vi "Joystick Driver Controls.vi"(4 "Shift Value":T1, 7 "X":dbl, 11 "Y":dbl) -> (2 "Y":dbl, 3 "X":dbl)   [LabVIEW 2016]
uses:
  <vilib>/Rock Robotics/WPI/Solenoid/WPI_SolenoidValue.ctl
  <vilib>/Rock Robotics/Network Tables/NT Read Number.vi
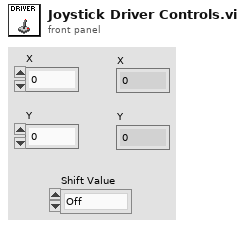
[diagram p1: front panel]
types:
  T1 = typedef "WPI_SolenoidValue.ctl" = enum16{"Off", "On", "Forward", "Reverse"}
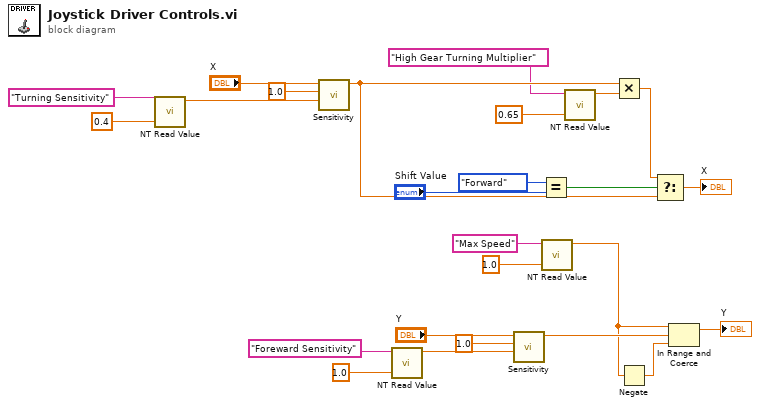
[diagram p0: block diagram]
diagram:
  n1 = call-poly <vilib>:"NT Read Value.vi"("Default Value"=0.4, "Name"="Turning Sensitivity") -> ("Numeric"=w7:dbl)  [unwired: 8 in, 1 out]
  n2 = call "Sensitivity.vi"("Power (z)"=w7, "Sensitivity (a)"=1.0, "Input"="X") -> ("Output"=w20:dbl)  [unwired: 8 in]
  n3 = call-poly <vilib>:"NT Read Value.vi"("Default Value"=1.0, "Name"="Foreward Sensitivity") -> ("Numeric"=w5:dbl)  [unwired: 8 in, 1 out]
  n4 = call "Sensitivity.vi"("Power (z)"=w5, "Sensitivity (a)"=1.0, "Input"="Y") -> ("Output"=w23:dbl)  [unwired: 8 in]
  n5 = Equal?(x=WPI_SolenoidValue."Forward", y="Shift Value") -> (x = y?=w15:bool)
  n6 = call-poly <vilib>:"NT Read Value.vi"("Default Value"=1.0, "Name"="Max Speed") -> ("Numeric"=w1:dbl)  [unwired: 8 in, 1 out]
  n7 = call-poly <vilib>:"NT Read Value.vi"("Default Value"=0.65, "Name"="High Gear Turning Multiplier") -> ("Numeric"=w10:dbl)  [unwired: 8 in, 1 out]
  n8 = Multiply(x=w20, y=w10) -> (x*y=w16:dbl)
  n9 = Negate(x=w1) -> (-x=w25:dbl)
  n10 = Select(t=w16, s=w15, f=w20) -> (s? t:f=→"X":dbl)
  n11 = In Range and Coerce(upper limit=w1, x=w23, lower limit=w25) -> (coerced(x)=→"Y":dbl)  [unwired: 1 out]
